vi "sprawdzRuchPionowy.vi"(8 "Wybór komory":T1, 9 "LINX Error IN":errorcluster, 10 "Czy nastapil krok?":bool, 11 "Stan pionowy":T2) -> (1 "LINX Error OUT":errorcluster, 2 "KONIEC":bool, 3 "Stan pionowy wybrany":T2)   [LabVIEW 2014]
uses:
  RuchPionowy.ctl
  parametryKomorVIs/WyborKomory.ctl
  poziomyVIs/timerRuchuPoziomegoVIs/Czynnosc.ctl
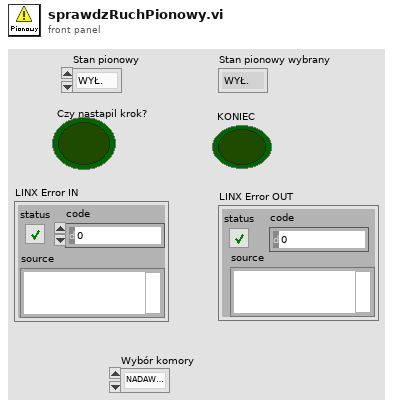
[diagram p1: front panel]
types:
  T1 = typedef "WyborKomory.ctl" = enum16{"NADAWCZA", "ODBIORCZA"}
  T2 = typedef "RuchPionowy.ctl" = enum16{"WYŁ.", "GÓRA", "Dӣ", "PRACA RĘCZNA"}
  T3 = typedef "Czynnosc.ctl" = enum16{"reset all", "działaj"}
  T4 = typedef "WejsciaParametry.ctl" = cluster{"LEWO":bool, "PRAWO":bool, "GORA":bool, "DOL":bool, "Praca reczna":bool, "Stop":bool, "Start":bool, "Komora":bool, "Wyjscie":bool, "Rodzaj pomiarow":T5, "Czas pomiaru [s]":dbl, "Czas inicjalizacji ramion [s]":dbl, "Liczba punktów":i32, "Liczba płaszczyzn":i32, "Komora nadawcza":bool, "Komora odbiorcza":bool}
  T5 = typedef "RodzajPomiarow.ctl" = enum16{"Izolacyjność Akustyczna ISO 10140", "Losowanie punktów", "Sekwencja testowa"}
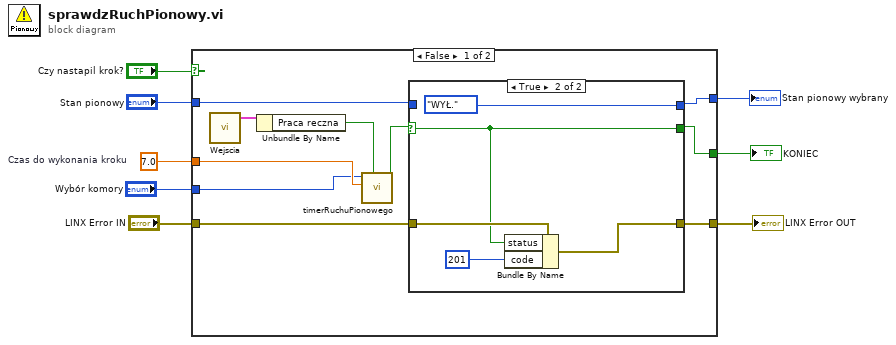
[diagram p0: block diagram]
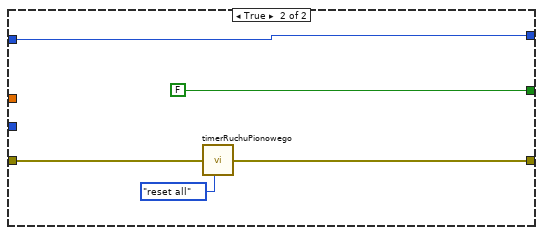
[diagram p3: hidden frame]
diagram:
  w7 = 7.0  # Czas do wykonania kroku
  n1 = case shown="False" "Czy nastapil krok?" {
    tunnel: "Stan pionowy" -> [w18 w30]
    tunnel: w7 -> [w15 _]
    tunnel: [w17 w30] -> w4
    tunnel: [w16 FALSE] -> w6
    tunnel: "LINX Error IN" -> [w13 w28]
    tunnel: [w12 w28] -> w2
    tunnel: "Wybór komory" -> [w11 _]
    frame False {
      n2 = call "Wejscia.vi"() -> ("Wyjście"=w10:T4)  [unwired: 5 in]
      n3 = Unbundle By Name(w10) -> ("Praca reczna"=w9:bool)
      n4 = call "timerRuchuPionowego.vi"("Pauza"=w9, "Czas"=w15, "Wybór komory"=w11) -> ("Czy czas upłynął?"=w14:bool)  [unwired: 8 in]
      n5 = case shown="True" w14 {
        selector: w14 -> [w20 w23]
        tunnel: w18 -> [w21 _]
        tunnel: [w21 RuchPionowy."WYŁ." ("Stan pionowy")] -> w17
        tunnel: [w20 w23] -> w16
        tunnel: w13 -> [w19 w24]
        tunnel: [w19 w22] -> w12
        frame False {
        }
        frame True {
          n6 = Bundle By Name(cluster=w24, "status"=w23, "code"=201 ("LINX Error Code")) -> (w22:errorcluster)
        }
      }
    }
    frame True {
      n7 = call "timerRuchuPionowego.vi"("Czynność"=Czynnosc."reset all") -> ()  [unwired: 10 in, 1 out]
    }
  }
  "KONIEC" <- w6
  "Stan pionowy wybrany" <- w4
  "LINX Error OUT" <- w2
